vi "CreateVerificationFile(Automatic).vi"   [LabVIEW 2019, in "Tools.lvlib"]
uses:
  Tools.lvlib
  ProjectPaths.ctl
panel:
  # "Run and DONE! :)"
types:
  T1 = typedef "Tools.lvlib/ProjectPaths.ctl" = enum16{"Settings dir", "Logs dir", "Resources dir", "Verification file", "Users file", "Root dir"}
  T2 = enum16{"open", "replace", "create", "open or create", "replace or create", "replace or create with confirmation"}
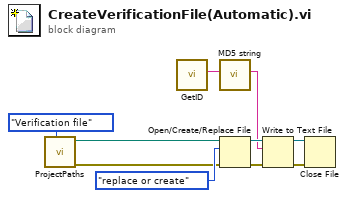
[diagram p0: block diagram]
diagram:
  n1 = call "ProjectPaths.vi"("Item"=ProjectPaths."Verification file") -> ("Error Out"=w2:errorcluster, "Path"=w3:path)  [unwired: 9 in]
  n2 = call "GetID.vi"() -> ("Computer ID"=w5:string)  [unwired: 10 in, 1 out]
  n3 = call "MD5 string.vi"("Message String"=w5) -> ("MD5 message-digest"=w4:string)  [unwired: 10 in]
  n4 = Open/Create/Replace File(file path (use dialog)=w3, error in=w2, operation (0:open)=T2."replace or create") -> (refnum out=w9:refnum<file>, error out=w8:errorcluster)  [unwired: 3 in, 1 out]
  n5 = Write to Text File(file (use dialog)=w9, text=w4, error in=w8) -> (refnum out=w6:refnum<file>, error out=w7:errorcluster)  [unwired: 1 in, 1 out]
  n6 = Close File(refnum=w6, error in=w7) -> ()  [unwired: 2 out]
